vi "HeartBeatDetectOffline1.vi"() -> ()   [LabVIEW 2014, in "Phonocardiography.lvlib"]
uses:
  <vilib>/Waveform/WDTOps.llb/WDT Index Channel DBL.vi
  <vilib>/Waveform/WDTOps.llb/WDT Get Waveform Time Array DBL.vi
  Phonocardiography.lvlib
  <vilib>/Analysis/NI_AAL_SigProc.lvlib
panel:
  in  "Remove\nEctopic Beats":bool=TRUE
  out "Heart rate":cluster{"X [s]":dbl[], "Heart Rate [BPM]":dbl[]}(graph)
  out "pNN50 [%]":dbl format="%0.2f"
  out "rMSSD  [ms]":dbl format="%0.2f"
  out "sdRR [ms]":dbl format="%0.2f"
  out "Mean RR [ms]":dbl format="%0.2f"
  out "Mean heart rate [BPM]":dbl
  out "Peaks":cluster{dbl[], "Amplitudes":dbl[]}[](graph)=[{array[122880 elements], "Amplitudes"=array[122880 elements]}, {[0.2683937704472721, 1.0181964328893598, 1.7377038104855096, 2.4855473692602947, 3.2774489982847803, 4.117602629900593, 5.0497054685009335, 5.994733213940523, 6.895302722768209, 7.797557321695085, 8.691660475532698, 9.53679206192987, 10.39302687835089], "Amplitudes"=[0.31315447076575686, 0.3206463592501255, 0.30828679771720463, 0.3046863092516966, 0.3208257168568248, 0.33907754062759177, 0.3184735631174685, 0.2664009802503432, 0.3439713540857765, 0.30399089060543044, 0.30335101069011816, 0.3364507699677884, 0.30464834692469883]}]
  in  "Negate":bool
  in  "Threshold mult":dbl=0.65 min=-1.0 max=1.0 step=0.05
  in  "width (threshold)":i32=30
  in  "File Path Control":path=path "C:/Users/Tamas/Documents/Projektek/Magzati szívhang/Nem babás/szep/nagy1.wav"
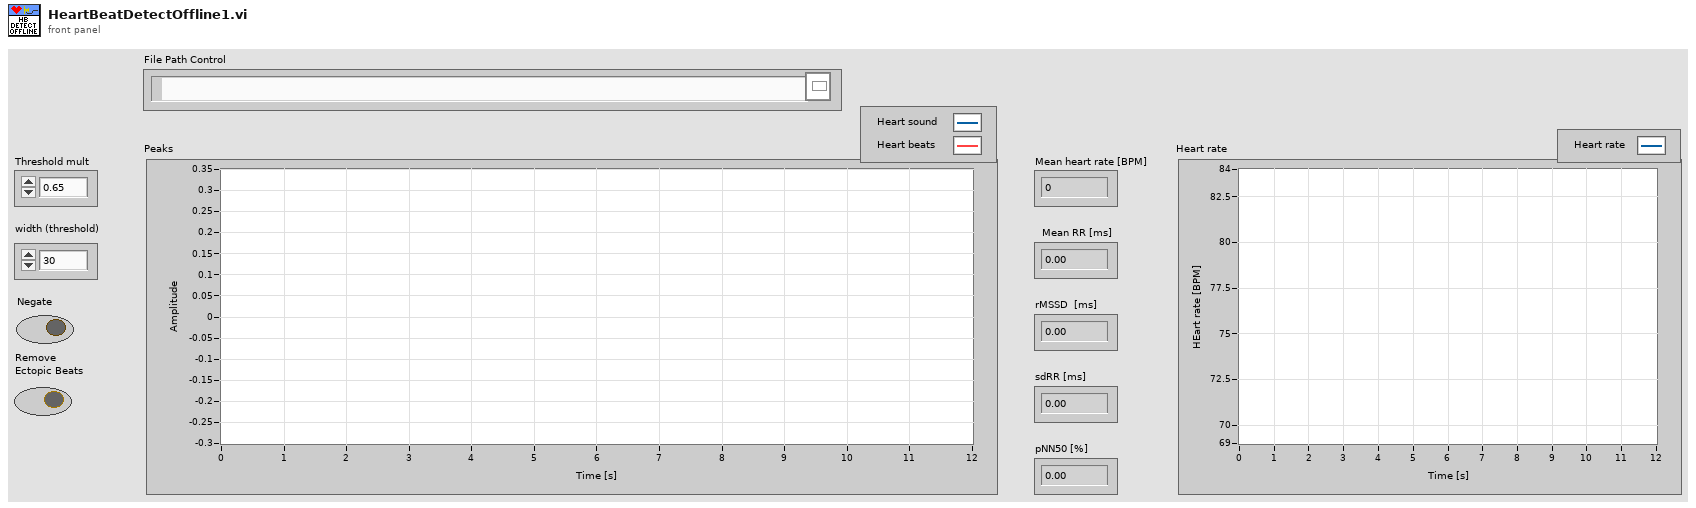
[diagram p1: front panel]
types:
  T1 = typedef "LVCursorListTypeDef.ctl" = cluster{"Name":string, "Color":u32, "Style":u8, "Point Style":u8, "Name Visible":bool, "Allow Drag":bool, "Cursor Mode":u32, "Plot":i32, "Index":i32, "Position":cluster{"X":dbl, "Y":dbl}, "X Scale":u32, "Y Scale":u32, "Watch Plots":i32[], "Watch All Plots":bool, "Plot Area":i32, "Label Offset":cluster{"X":dbl, "Y":dbl}}[]
  T2 = cluster{"Name":string, "Color":u32, "Style":u8, "Point Style":u8, "Name Visible":bool, "Allow Drag":bool, "Cursor Mode":u32, "Plot":i32, "Index":i32, "Position":cluster{"X":dbl, "Y":dbl}, "X Scale":u32, "Y Scale":u32, "Watch Plots":i32[], "Watch All Plots":bool, "Plot Area":i32, "Label Offset":cluster{"X":dbl, "Y":dbl}}
  T3 = cluster{"Name":string, "Color":u32, "Style":u8, "Point Style":u8, "Name Visible":bool, "Allow Drag":bool, "Cursor Mode":u32, "Plot":i32, "Index":i32, "Position":cluster{"X":dbl, "Y":dbl}, "X Scale":u32, "Y Scale":u32, "Watch Plots":i32[], "Watch All Plots":bool, "Plot Area":i32, "Label Offset":cluster{"X":dbl, "Y":dbl}}[]
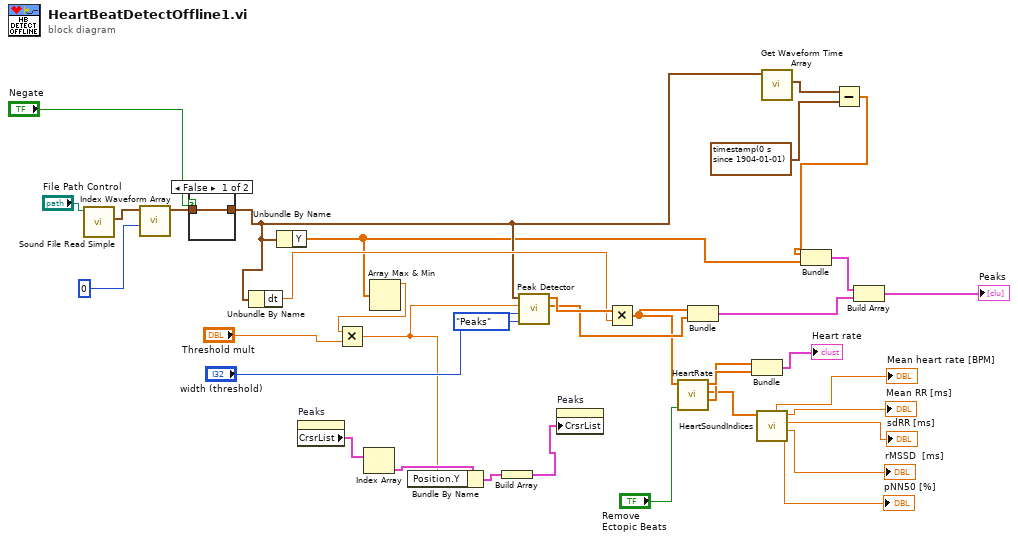
[diagram p0: block diagram]
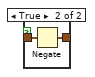
[diagram p2: hidden frame]
diagram:
  n1 = call <vilib>:"Sound File Read Simple.vi"("path"="File Path Control") -> ("data"=w35:waveform(dbl)[])  [unwired: 7 in, 3 out]
  n2 = call-poly <vilib>:"Index Waveform Array.vi"("index"=0, "waveform array"=w35) -> ("waveform"=w31:waveform(dbl))  [unwired: 8 in, 1 out]
  n3 = case shown="False" "Negate" {
    tunnel: w31 -> [w37 w39]
    tunnel: [w37 w38] -> w16
    frame False {
    }
    frame True {
      n4 = Negate(x=w39) -> (-x=w38:waveform(dbl))
    }
  }
  n5 = Unbundle By Name(w16) -> ("dt"=w23:dbl)
  n6 = Unbundle By Name(w16) -> ("Y"=w14:dbl[])
  n7 = property on="Peaks" class="XYGraph (strict)"() -> ("CrsrList"=w20:T1)  [unwired: 2 in, 2 out]
  n8 = Index Array(array=w20) -> (element=w29:T2)  [unwired: 1 in]
  n9 = Array Max & Min(array=w14) -> (max value=w28:dbl)  [unwired: 3 out]
  n10 = Multiply(x=w28, y="Threshold mult") -> (x*y=w25:dbl)
  n11 = Bundle By Name(cluster=w29, "Position.Y"=w25) -> (w27:T2)
  n12 = Build Array(w27) -> (w19:T3)
  n13 = call <vilib>:"Peak Detector.vi"("peaks/valleys"=enum32{"Peaks", "Valleys"}."Peaks", "width"="width (threshold)", "threshold"=w25, "X"=w16) -> ("Amplitudes"=w22:dbl[], "Locations"=w24:dbl[])  [unwired: 3 in, 3 out]
  n14 = property on="Peaks" class="XYGraph (strict)"("CrsrList"=w19) -> ()  [unwired: 2 in, 2 out]
  n15 = Multiply(x=w24, y=w23) -> (x*y=w11:dbl[])
  n16 = call "HeartRate.vi"("Remove Ectopic?"="Remove\nEctopic Beats", "Peaks X in"=w11) -> ("X [s]"=w9:dbl[], "RR intervals [ms]"=w8:dbl[], "Heart Rate [BPM]"=w10:dbl[])  [unwired: 7 in]
  n17 = Bundle(w11, "Amplitudes"=w22) -> (w32:cluster{dbl[], "Amplitudes":dbl[]})  [unwired: 1 in]
  n18 = Bundle("X [s]"=w9, "Heart Rate [BPM]"=w10) -> (→"Heart rate":cluster{"X [s]":dbl[], "Heart Rate [BPM]":dbl[]})  [unwired: 1 in]
  n19 = call "HeartSoundIndices.vi"("RR intervals [ms]"=w8) -> ("pNN50 [%]"=→"pNN50 [%]":dbl, "rMSSD  [ms]"=→"rMSSD  [ms]":dbl, "sdRR [ms]"=→"sdRR [ms]":dbl, "Mean RR [ms]"=→"Mean RR [ms]":dbl, "Mean heart rate [BPM]"=→"Mean heart rate [BPM]":dbl)  [unwired: 6 in]
  n20 = call-poly <vilib>:"Get Waveform Time Array.vi"("waveform in"=w16) -> ("X array"=w18:timestamp[])  [unwired: 9 in, 1 out]
  n21 = Subtract(x=w18, y=timestamp(0 s since 1904-01-01) ("Xo")) -> (x-y=w15:dbl[])
  n22 = Bundle(w15, "Y"=w14) -> (w13:cluster{dbl[], "Y":dbl[]})  [unwired: 1 in]
  n23 = Build Array(w13, w32) -> (→"Peaks":cluster{dbl[], "Amplitudes":dbl[]}[])
